vi "Point to Row And Col.vi"(8 "错误输入（无错误）":errorcluster, 10 "点":T2, 11 "Ref":refnum<vi>) -> (0 "错误输出":errorcluster, 2 "Point to Row and Col":cluster{"单元格位置":T1, "边界内？":bool, "符号内？":bool}, 3 "Dup Ref":refnum<vi>)   [LabVIEW 2012, in "Mlistbox Tools.lvlib"]
uses:
  Mlistbox Tools.lvlib
  <vilib>/Utility/miscctls.llb/LVPositionTypeDef.ctl
  <vilib>/Utility/miscctls.llb/LVRowAndColumnTypeDef.ctl
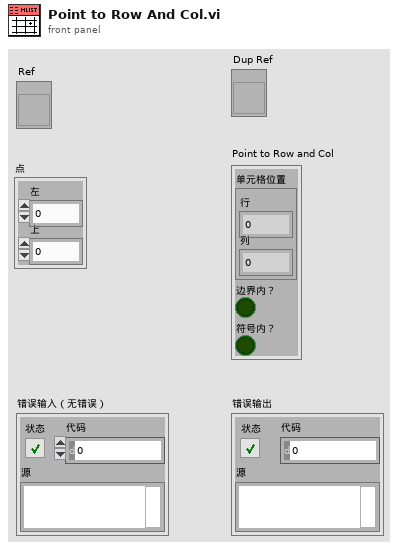
[diagram p1: front panel]
types:
  T1 = typedef "LVRowAndColumnTypeDef.ctl" = cluster{"Row":i32, "Column":i32}
  T2 = typedef "LVPositionTypeDef.ctl" = cluster{"Left":i32, "Top":i32}
  T3 = cluster{"CellPosition":T1, "InBounds":bool, "InGlyph":bool}
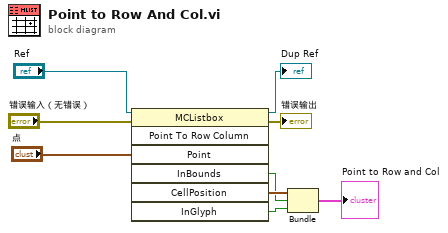
[diagram p0: block diagram]
diagram:
  n1 = invoke on="调用节点" class="MCListbox" method="Point To Row Column"(reference="Ref", error in="错误输入（无错误）", "Point"="点") -> (reference out=→"Dup Ref":refnum<vi>, error out=→"错误输出":errorcluster, "InBounds"=w3:bool, "CellPosition"=w4:T1, "InGlyph"=w2:bool)  [unwired: 4 in, 2 out]
  n2 = Bundle("CellPosition"=w4, "InBounds"=w3, "InGlyph"=w2) -> (→"Point to Row and Col":T3)  [unwired: 1 in]
